vi "GetText.vi"(8 "error in":errorcluster, 11 "current in":refnum<class "Current.lvclass">) -> (0 "error out":errorcluster, 1 "additional text":string, 2 "text":string, 3 "current out":refnum<class "Current.lvclass">, 4 "glyph":string)   [LabVIEW 2013, in "Current.lvclass"]
uses:
  Current.lvclass
  Channel/Channel.lvclass
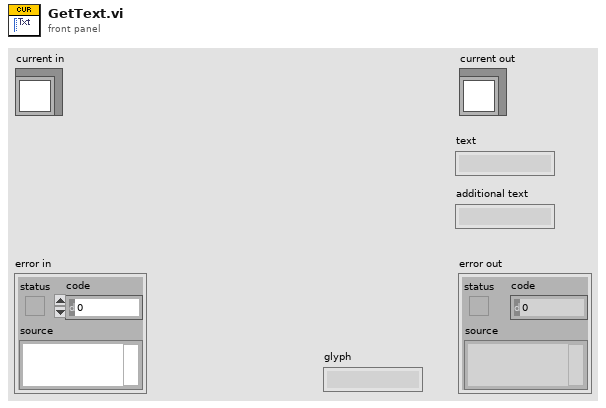
[diagram p1: front panel]
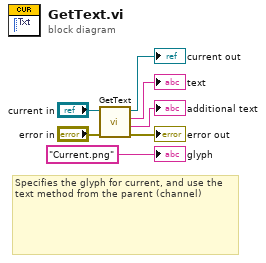
[diagram p0: block diagram]
diagram:
  # "Specifies the glyph for current, and use the text method from the parent (channel)"
  n1 = call-parent "GetText.vi"("error in"="error in", "channel in"="current in") -> ("error out"=→"error out":errorcluster, "additional text"=→"additional text":string, "text"=→"text":string, "channel out"=→"current out":refnum<class "Current.lvclass">)  [unwired: 5 in, 1 out]
  "glyph" <- "Current.png" ("glyph")
